vi "Adaptador de datos.vi"(6 "Cant. de pulsos":u16, 7 "Reduccion":sgl, 8 "error in (no error)":errorcluster, 9 "Encoder":u16, 10 "Transductores":u16[](array[numeric])) -> (0 "error out":errorcluster, 2 "Encoder":sgl, 3 "Transductores":sgl[](array[numeric]))   [LabVIEW 2014, in "CAP-USB.lvlib"]
doc: "VI encargado del escalamiento de los datos de entrada por parte del CAP-USB1.0"
uses:
  CAP-USB.lvlib
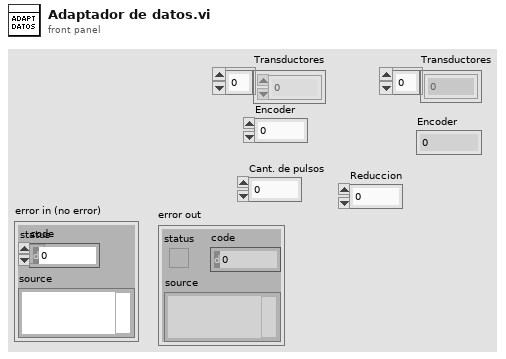
[diagram p1: front panel]
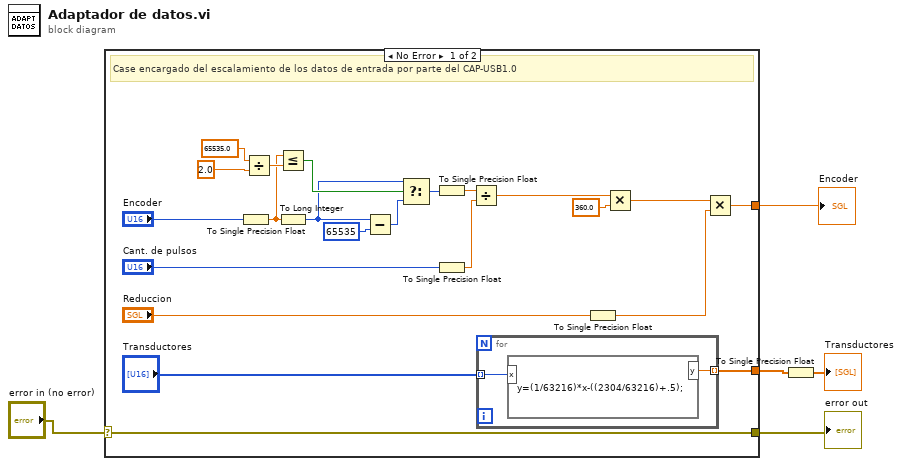
[diagram p0: block diagram]
diagram:
  n1 = case shown="No Error" "error in (no error)" {
    selector: "error in (no error)" -> [w27 w30]
    tunnel: [w27 w30] -> w5
    tunnel: [w25 _] -> w4
    tunnel: [w18 _] -> w1
    frame No Error {
      # "Case encargado del escalamiento de los datos de entrada por parte del CAP-USB1.0"
      n2 = To Single Precision Float(number="Encoder") -> (single precision float=w6:sgl)
      n3 = Divide(x=sgl 65535.0, y=sgl 2.0) -> (x/y=w8:sgl)
      n4 = Less Or Equal?(x=w6, y=w8) -> (x <= y?=w17:bool)
      n5 = To Long Integer(number=w6) -> (32bit integer=w14:i32)
      n6 = Subtract(x=w14, y=65535) -> (x-y=w15:i32)
      n7 = Select(t=w14, s=w17, f=w15) -> (s? t:f=w23:i32)
      n8 = To Single Precision Float(number=w23) -> (single precision float=w24:sgl)
      n9 = To Single Precision Float(number="Cant. de pulsos") -> (single precision float=w21:sgl)
      n10 = Divide(x=w24, y=w21) -> (x/y=w13:sgl)
      n11 = for {
        tunnel: "Transductores" -> [w29] mode=indexing
        tunnel: [w28] -> w25 mode=indexing
        n12 = formula code="y=(1/63216)*x-((2304/63216)+.5);"("x"=w29) -> ("y"=w28:dbl)
      }
      n13 = To Single Precision Float(number="Reduccion") -> (single precision float=w19:sgl)
      n14 = Multiply(x=w13, y=sgl 360.0) -> (x*y=w12:sgl)
      n15 = Multiply(x=w12, y=w19) -> (x*y=w18:sgl)
    }
    frame Error {
    }
  }
  "Encoder" <- w1
  "error out" <- w5
  n16 = To Single Precision Float(number=w4) -> (single precision float=→"Transductores":sgl[])
